vi "Try Consume Modifier Token.vi"(11 "Pattern Parser In":T3) -> (1 "Null?":bool, 2 "Token":T1, 3 "Pattern Parser":T3)   [LabVIEW 2020, in "Stream.lvlib" / "URLPattern.lvclass"]
uses:
  URLPattern.lvclass
  Pattern Parser.ctl
  Token.ctl
  Token Type.ctl
  Pattern Part.ctl
  Pattern Part Type.ctl
  Pattern Part Modifier.ctl
  Token Type Equals.vi
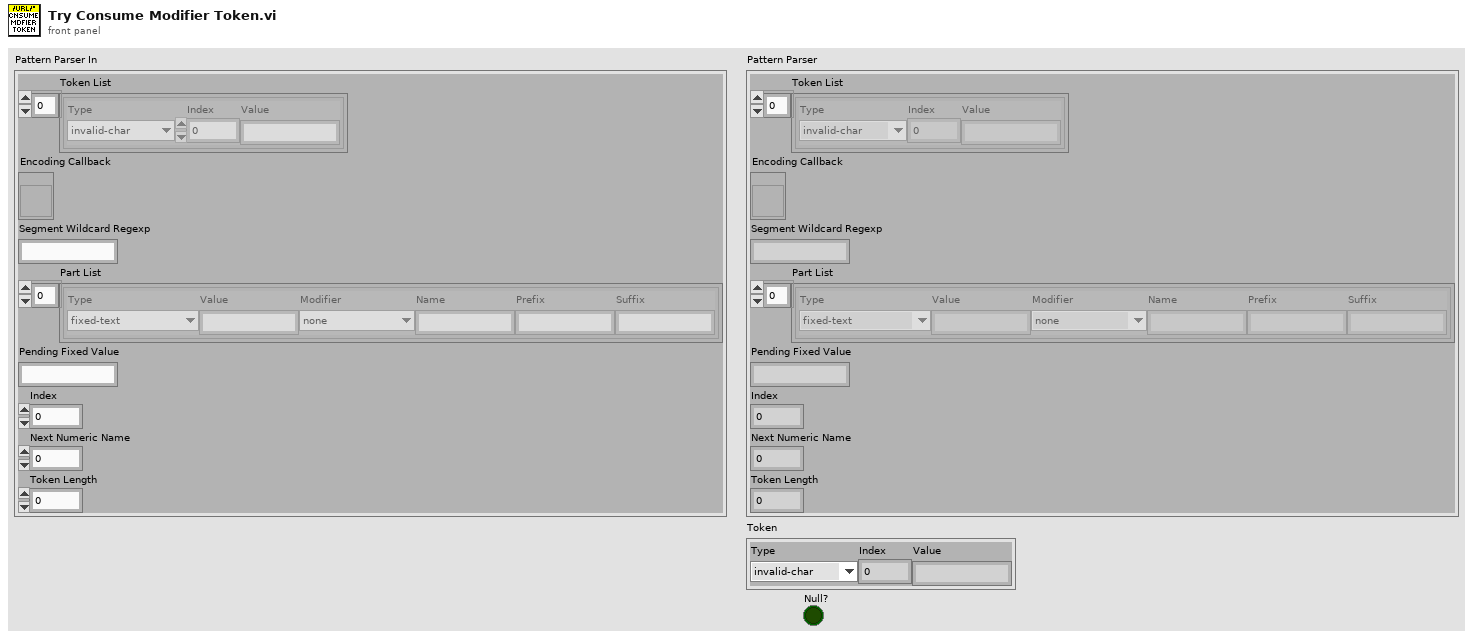
[diagram p1: front panel]
types:
  T1 = typedef "Stream.lvlib/URLPattern.lvclass/Token.ctl" = cluster{"Type":T2, "Index":i32, "Value":string}
  T2 = typedef "Stream.lvlib/URLPattern.lvclass/Token Type.ctl" = enum16{"invalid-char", "open", "close", "regexp", "name", "char", "escaped-char", "other-modifier", "asterisk", "end"}
  T3 = typedef "Stream.lvlib/URLPattern.lvclass/Pattern Parser.ctl" = cluster{"Token List":T1[], "Encoding Callback":refnum<vi>, "Segment Wildcard Regexp":string, "Part List":T4[], "Pending Fixed Value":string, "Index":i32, "Next Numeric Name":i32, "Token Length":i32}
  T4 = typedef "Stream.lvlib/URLPattern.lvclass/Pattern Part.ctl" = cluster{"Type":T5, "Value":string, "Modifier":T6, "Name":string, "Prefix":string, "Suffix":string}
  T5 = typedef "Stream.lvlib/URLPattern.lvclass/Pattern Part Type.ctl" = enum16{"fixed-text", "regexp", "segment-wildcard", "full-wildcard"}
  T6 = typedef "Stream.lvlib/URLPattern.lvclass/Pattern Part Modifier.ctl" = enum16{"none", "optional", "zero-or-more", "one-or-more"}
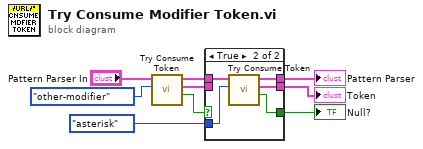
[diagram p0: block diagram]
diagram:
  n1 = call "Try Consume Token.vi"("Type"=Token_Type."other-modifier", "Pattern Parser In"="Pattern Parser In") -> ("Null?"=w7:bool, "Token"=w5:T1, "Pattern Parser"=w6:T3)  [unwired: 7 in]
  n2 = case shown="True" w7 {
    selector: w7 -> [w10 _]
    tunnel: w6 -> [w12 w17]
    tunnel: w5 -> [w11 _]
    tunnel: [w12 w15] -> w4
    tunnel: [w11 w14] -> w3
    tunnel: [w10 w13] -> w2
    tunnel: Token_Type."asterisk" ("Type") -> [_ w16]
    frame False {
    }
    frame True {
      n3 = call "Try Consume Token.vi"("Type"=w16, "Pattern Parser In"=w17) -> ("Null?"=w13:bool, "Token"=w14:T1, "Pattern Parser"=w15:T3)  [unwired: 7 in]
    }
  }
  "Pattern Parser" <- w4
  "Token" <- w3
  "Null?" <- w2
